vi "Set Multicast Endpoint.vi"(8 "error in (no error)":errorcluster, 10 "Multicast Endpoint":T1, 11 "Group in":refnum<class "Group Config.lvclass">) -> (0 "error out":errorcluster, 3 "Group out":refnum<class "Group Config.lvclass">)   [LabVIEW 2020, in "VolatusConfig.lvlib" / "Group Config.lvclass"]
uses:
  Group Config.lvclass
  C:/dev/lv20CE/relink/lv-volatus/VolatusConfig/VolatusConfigElement/VolatusConfigElement.lvclass
  lv-vecto/VectoConfig/Endpoint.ctl
  lv-cdm/CDM-Config/Value Type.ctl
  VolatusConfigElement/VolatusConfigElement.lvclass/VolatusConfigElement.ctl
  lv-cdm/CDM-Config/Config Element/Write Variant Value.vi
  Group Config.lvclass/Group Config.ctl
  lv-cdm/CDM-Config/Config Element/Config Element.lvclass
  VolatusConfigElement/VolatusConfigElement.lvclass
  lv-cdm/CDM-Config/CDM-Config.lvlib
  lv-vecto/VectoConfig/VectoConfig.lvlib
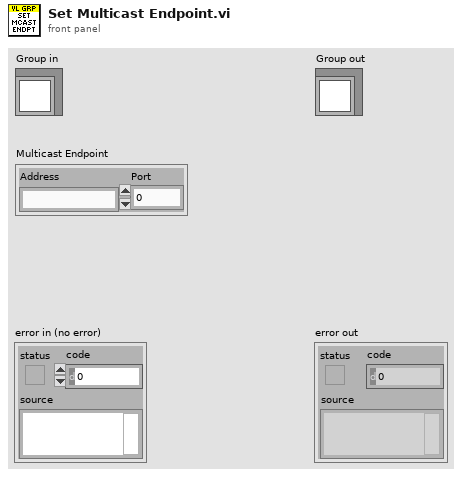
[diagram p1: front panel]
types:
  T1 = typedef "VectoConfig.lvlib/Endpoint.ctl" = cluster{"Address":string, "Port":u16}
  T2 = typedef "CDM-Config.lvlib/Value Type.ctl" = enum16{"String", "Number", "Bool", "Object", "Array"}
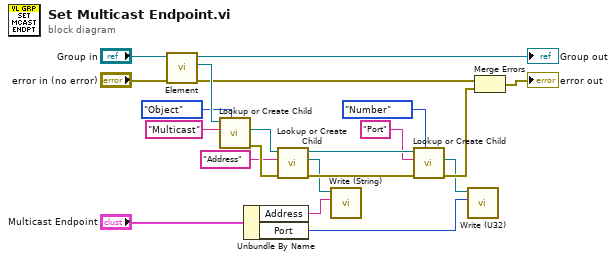
[diagram p0: block diagram]
diagram:
  n1 = call "Element.vi"("VolatusConfigElement in"="Group in") -> ("Element"=w18:refnum<class "Config Element.lvclass">, "VolatusConfigElement out"=→"Group out":refnum<class "Group Config.lvclass">)  [unwired: 9 in]
  n2 = call "Lookup or Create Child.vi"("Value Type (Object)"=Value_Type."Object" ("Value Type (String)"), "Name"="Multicast", "Config Element in"=w18) -> ("error out"=w19:errorcluster, "Child"=w15:refnum<class "Config Element.lvclass">)  [unwired: 5 in, 2 out]
  n3 = Unbundle By Name("Multicast Endpoint") -> ("Address"=w8:string, "Port"=w6:u16)
  n4 = call "Lookup or Create Child.vi"("error in (no error)"=w19, "Name"="Address", "Config Element in"=w15) -> ("error out"=w12:errorcluster, "Child"=w9:refnum<class "Config Element.lvclass">, "Config Element out"=w13:refnum<class "Config Element.lvclass">)  [unwired: 5 in, 1 out]
  n5 = call "Write (String).vi"("String Value"=w8, "Config Element in"=w9) -> ()  [unwired: 8 in, 2 out]
  n6 = call "Lookup or Create Child.vi"("Value Type (Object)"=Value_Type."Number" ("Value Type (String)"), "error in (no error)"=w12, "Name"="Port", "Config Element in"=w13) -> ("error out"=w20:errorcluster, "Child"=w7:refnum<class "Config Element.lvclass">)  [unwired: 4 in, 2 out]
  n7 = call "Write (U32).vi"("U32 Value"=w6, "Config Element in"=w7) -> ()  [unwired: 8 in, 2 out]
  n8 = Merge Errors("error in (no error)", w20) -> (→"error out":errorcluster)
